vi "Open Folder.vi"(8 "Error in (no error)":errorcluster, 11 "Controller in":refnum<class "Controller.lvclass">) -> (0 "Error out":errorcluster, 3 "Controller out":refnum<class "Controller.lvclass">)   [LabVIEW 2022 SP3, in "Controller.lvlib" / "Controller.lvclass"]
uses:
  Controller.lvclass
  Controller.lvclass/Controller.ctl
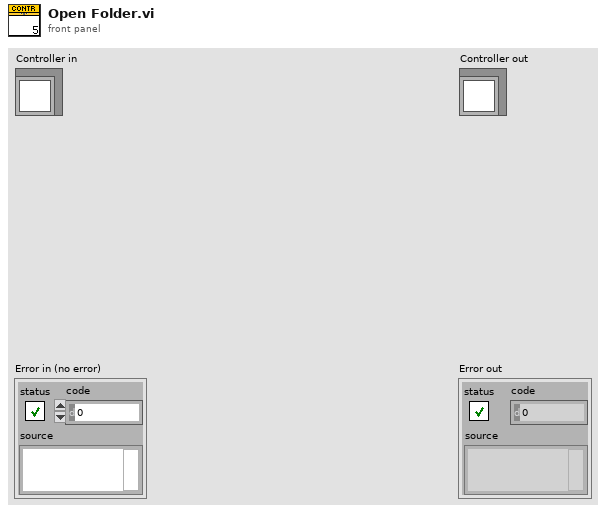
[diagram p1: front panel]
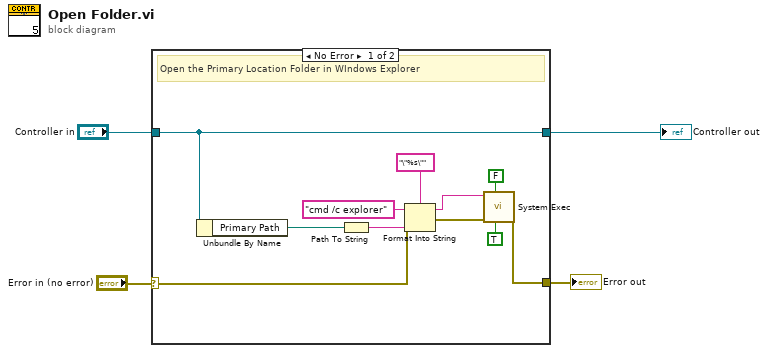
[diagram p0: block diagram]
diagram:
  n1 = case shown="No Error" "Error in (no error)" {
    selector: "Error in (no error)" -> [w6 w17]
    tunnel: "Controller in" -> [w5 w16]
    tunnel: [w7 w17] -> w3
    tunnel: [w5 w16] -> w1
    frame No Error {
      # "Open the Primary Location Folder in WIndows Explorer"
      n2 = Unbundle By Name(w5) -> ("Primary Path"=w15:path)
      n3 = Path To String(path=w15) -> (string=w14:string)
      n4 = Format Into String(format string="\"%s\"", initial string="cmd /c explorer", error in=w6, w14) -> (resulting string=w11:string, error out=w10:errorcluster)
      n5 = call <vilib>:"System Exec.vi"("run minimized? (F)"=TRUE, "wait until completion? (T)"=FALSE, "error in (no error)"=w10, "command line"=w11) -> ("error out"=w7:errorcluster)  [unwired: 4 in, 3 out]
    }
    frame Error {
    }
  }
  "Error out" <- w3
  "Controller out" <- w1
